vi "TestPFGVReadUIDs.vi"() -> (0 "error out":errorcluster, 2 "Pass":bool)   [LabVIEW 2015]
uses:
  TypeDef/PersonnelActions.ctl
panel:
  out "PUIDs Init":string
  out "PUIDs Personnel":string
  in  "PUID":string="d1"
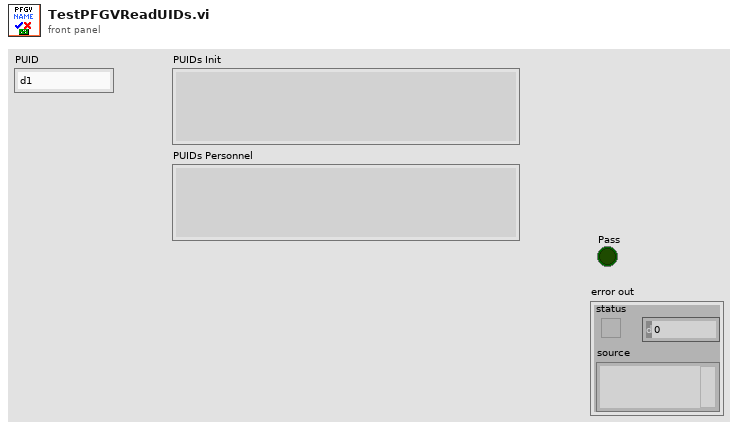
[diagram p1: front panel]
types:
  T1 = typedef "PersonnelActions.ctl" = enum16{"Init", "Read Personnel", "Add Personnel", "Remove Personnel", "Read Name", "Write Name", "Read Role", "Write Role", "Read Requests", "Add Requests", "Remove Requests", "Read PUIDs"}
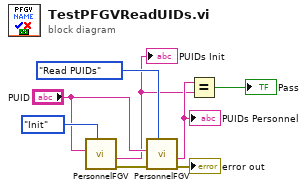
[diagram p0: block diagram]
diagram:
  n1 = call "PersonnelFGV.vi"("Actions"=PersonnelActions."Init", "PUID"="PUID") -> ("error out"=w8:errorcluster, "Data Out"=w2:string)  [unwired: 8 in]
  "PUIDs Init" <- w2
  n2 = call "PersonnelFGV.vi"("Actions"=PersonnelActions."Read PUIDs", "error in (no error)"=w8, "PUID"="PUID") -> ("error out"=→"error out":errorcluster, "Data Out"=w3:string)  [unwired: 7 in]
  "PUIDs Personnel" <- w3
  n3 = Equal?(x=w3, y=w2) -> (x = y?=→"Pass":bool)
